vi "Get Data Value.vi"(8 "error in (no error)":errorcluster, 11 "numericPayload in":refnum<class "numericPayload.lvclass">) -> (0 "error out":errorcluster, 1 "Data Value out":dbl, 3 "numericPayload out":refnum<class "numericPayload.lvclass">)   [LabVIEW 2017, in "messagesPayload.lvlib" / "numericPayload.lvclass"]
uses:
  numericPayload.lvclass
  numericPayload.lvclass/numericPayload.ctl
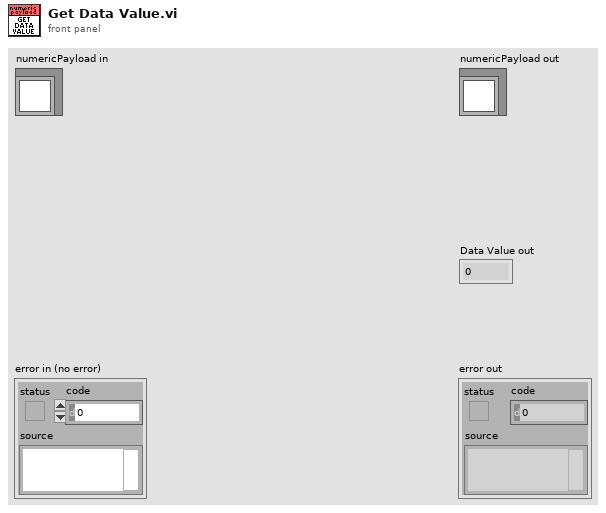
[diagram p1: front panel]
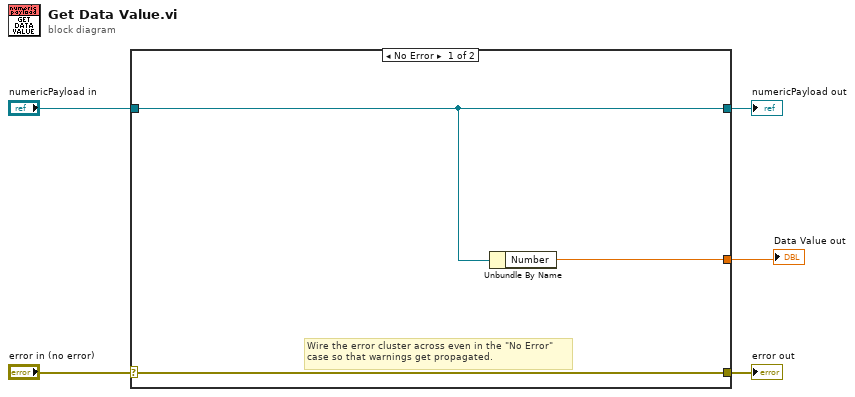
[diagram p0: block diagram]
diagram:
  n1 = case shown="No Error" "error in (no error)" {
    selector: "error in (no error)" -> [w8 w10]
    tunnel: [w8 w10] -> w4
    tunnel: [w6 w9] -> w2
    tunnel: "numericPayload in" -> [w6 w9]
    tunnel: [w7 _] -> w1
    frame No Error {
      # "Wire the error cluster across even in the \"No Error\"\ncase so that warnings get propagated."
      n2 = Unbundle By Name(w6) -> ("Number"=w7:dbl)
    }
    frame Error {
    }
  }
  "error out" <- w4
  "numericPayload out" <- w2
  "Data Value out" <- w1
